vi "Decoder.vi"(8 "error in (no error)":errorcluster, 11 "ISO 14443 B DOWN in":refnum<class "ISO 14443 B DOWN.lvclass">) -> (0 "error out":errorcluster, 3 "ISO 14443 B DOWN out":refnum<class "ISO 14443 B DOWN.lvclass">)   [LabVIEW 2019, in "ISO 14443 B DOWN.lvclass"]
uses:
  ISO 14443 B DOWN.lvclass
  TypeDef/Store.ctl
  ISO 14443 B DOWN.lvclass/ISO 14443 B DOWN.ctl
  RFID system.lvclass
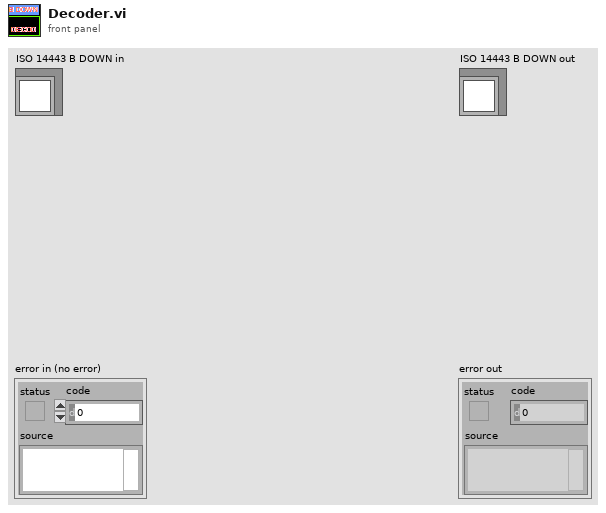
[diagram p1: front panel]
types:
  T1 = typedef "Store.ctl" = enum16{"envelope", "noise", "demSubCar", "CH_frame", "Decode", "demodulate", "in", "out", "sum", "subCarrier", "frame", "command", "encode", "modulate", "encode_UP", "modulate_up", "demod_up", "envelop_up", "sum_up", "out_up", "in_up"}
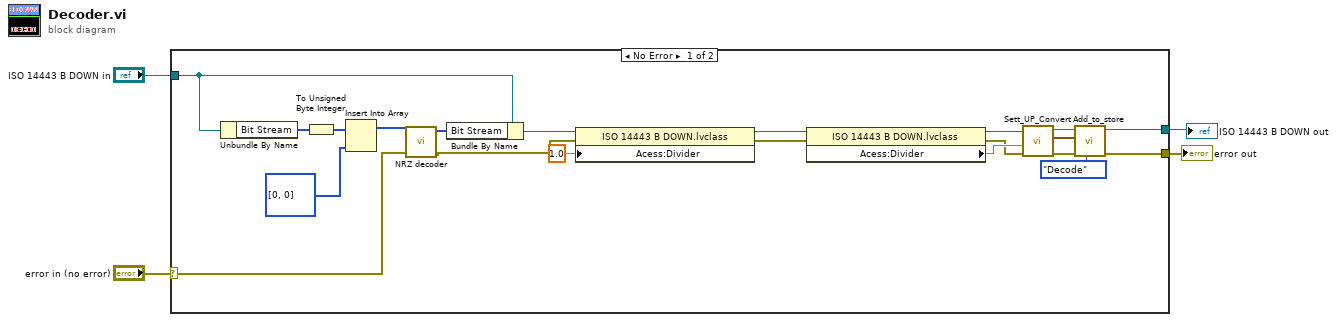
[diagram p0: block diagram]
diagram:
  n1 = case shown="No Error" "error in (no error)" {
    selector: "error in (no error)" -> [w8 w27]
    tunnel: [w18 w27] -> w1
    tunnel: "ISO 14443 B DOWN in" -> [w22 w26]
    tunnel: [w19 w26] -> w2
    frame No Error {
      n2 = Unbundle By Name(w22) -> ("Bit Stream"=w23:u8[])
      n3 = To Unsigned Byte Integer(number=w23) -> (unsigned 8bit integer=w25:u8[])
      n4 = Insert Into Array(array=w25, new element=u8[] [0, 0]) -> (w6:u8[])  [unwired: 1 in]
      n5 = call "NRZ decoder.vi"("error in (no error)"=w8, "Bit stream in"=w6) -> ("error out"=w7:errorcluster, "Array"=w5:u8[])  [unwired: 8 in]
      n6 = Bundle By Name(cluster=w22, "Bit Stream"=w5) -> (w21:refnum<class "ISO 14443 B DOWN.lvclass">)
      n7 = property class="ISO 14443 B DOWN.lvclass"(reference=w21, error in=w7, "Acess:Divider"=1.0 ("Divider")) -> (reference out=w11:refnum<class "ISO 14443 B DOWN.lvclass">, error out=w10:errorcluster)
      n8 = property class="ISO 14443 B DOWN.lvclass"(reference=w11, error in=w10) -> (reference out=w14:refnum<class "ISO 14443 B DOWN.lvclass">, error out=w12:errorcluster, "Acess:Divider"=w13:dbl)
      n9 = call-dynamic "Sett_UP_Convert.vi"("error in (no error)"=w12, "Divider(1)"=w13, "ISO 14443 B DOWN in"=w14) -> ("error out"=w17:errorcluster, "Waveform"=w16:waveform(dbl), "ISO 14443 B DOWN out"=w20:refnum<class "ISO 14443 B DOWN.lvclass">)  [unwired: 6 in]
      n10 = call "Add_to_store.vi"("Store"=Store."Decode", "error in (no error)"=w17, "Waveform"=w16, "RFID system in"=w20) -> ("error out"=w18:errorcluster, "RFID system out"=w19:refnum<class "ISO 14443 B DOWN.lvclass">)  [unwired: 6 in]
    }
    frame Error {
    }
  }
  "error out" <- w1
  "ISO 14443 B DOWN out" <- w2
